vi "3-revised.vi"() -> ()   [LabVIEW 2021]
uses:
  <vilib>/gmath/NI_AAL_MathFunc.lvlib
panel:
  out "Number 2":i32
  in  "Number":u64
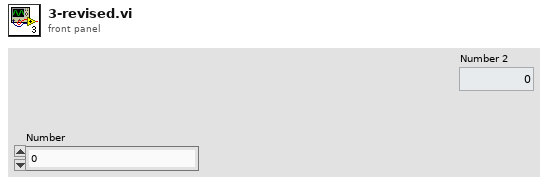
[diagram p1: front panel]
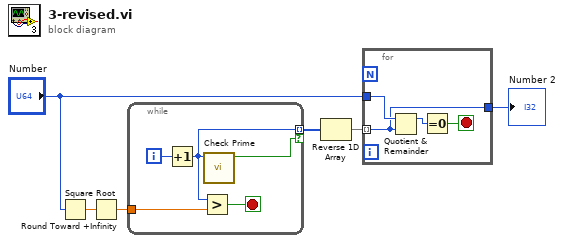
[diagram p0: block diagram]
diagram:
  n1 = Square Root(x="Number") -> (sqrt(x)=w6:dbl)
  n2 = Round Toward +Infinity(x=w6) -> (ceil(x): smallest int >= x=w5:dbl)
  n3 = while {
    tunnel: w5 -> [w10]
    tunnel: [w8] -> w4 mode=indexing if=w7
    i -> [w11]
    stop <- w9 stop-if-true
    n4 = Increment(x=w11) -> (x+1=w8:i32)
    n5 = Greater?(x=w8, y=w10) -> (0:w9:bool)
    n6 = call <vilib>:"Check Prime.vi"("n"=w8) -> ("prime?"=w7:bool)  [unwired: 10 in]
  }
  n7 = Reverse 1D Array(array=w4) -> (reversed array=w3:i32[])
  n8 = for {
    tunnel: w3 -> [w12] mode=indexing
    tunnel: "Number" -> [w13]
    tunnel: [w12] -> w2
    stop <- w14 stop-if-true
    n9 = Quotient & Remainder(x=w13, y=w12) -> (x-y*floor(x/y)=w15:u64)  [unwired: 1 out]
    n10 = Equal To 0?(x=w15) -> (x = 0?=w14:bool)
  }
  "Number 2" <- w2
